vi "DAC_set_slot-trigger.vi"(8 "Stop":bool, 9 "Cluster":T1, 10 "slot number":u16, 11 "FPGA VI Reference In":T2) -> (3 "FPGA VI Reference Out":T2)   [LabVIEW 2013]
uses:
  fpga-bitfile-ref.ctl
  slot-use-values.ctl
  slot-use-type.ctl
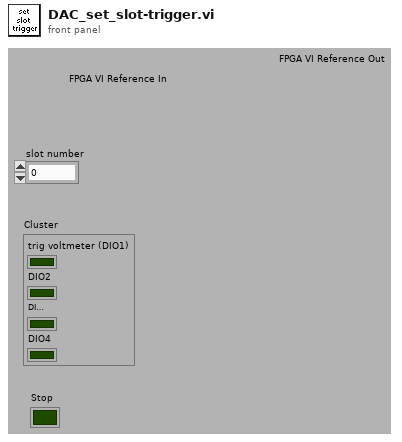
[diagram p1: front panel]
types:
  T1 = cluster{"trig voltmeter (DIO1)":bool, "DIO2":bool, "DIO3":bool, "DIO4":bool}
  T2 = typedef "fpga-bitfile-ref.ctl" = refnum<k20>
  T3 = typedef "slot-use-type.ctl" = fxp<+,4,4>
  T4 = typedef "slot-use-values.ctl" = enum16{"DAC", "timing", "triggers", "jump"}
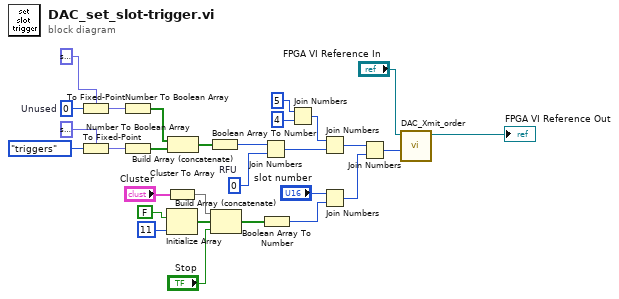
[diagram p0: block diagram]
diagram:
  w13 = u8 0  # Unused
  w26 = u8 0  # RFU
  n1 = To Fixed-Point(fixed-point type=T3 0.0, number=w13) -> (fixed-point=w18:T3)
  n2 = To Fixed-Point(fixed-point type=T3 0.0, number=slot-use-values."triggers") -> (fixed-point=w17:T3)
  n3 = Number To Boolean Array(number=w18) -> (Boolean array=w1:bool[])
  n4 = Number To Boolean Array(number=w17) -> (Boolean array=w2:bool[])
  n5 = Cluster To Array(cluster="Cluster") -> (array=w3:bool[])
  n6 = Initialize Array(FALSE ("1"), 11 ("taille de la dimension")) -> (w10:bool[])
  n7 = Build Array (concatenate)(w1, w2) -> (w19:bool[])
  n8 = Boolean Array To Number(Boolean array=w19) -> (number=w11:u8)
  n9 = Build Array (concatenate)(w3, w10, "Stop") -> (w7:bool[])
  n10 = Join Numbers(hi=w11, lo=w26) -> ((hi.lo)=w25:u16)
  n11 = Boolean Array To Number(Boolean array=w7) -> (number=w6:u16)
  n12 = Join Numbers(hi=u8 5, lo=u8 4) -> ((hi.lo)=w24:u16)
  n13 = Join Numbers(hi=w24, lo=w25) -> ((hi.lo)=w21:u32)
  n14 = Join Numbers(hi="slot number", lo=w6) -> ((hi.lo)=w22:u32)
  n15 = Join Numbers(hi=w21, lo=w22) -> ((hi.lo)=w29:u64)
  n16 = call "DAC_Xmit_order.vi"("Order in"=w29, "FPGA VI Reference In"="FPGA VI Reference In") -> ("FPGA VI Reference Out"=→"FPGA VI Reference Out":T2)  [unwired: 9 out]
